vi "Create Mecanum Steering Frame.vi"(8 "error in (no error)":errorcluster, 9 "wheel separation length":dbl=1.5, 10 "wheel separation width":dbl=1.0, 11 "wheels":T1) -> (0 "error out":errorcluster, 3 "mecanum steering frame out":refnum<class "NI_Robotics_Mecanum Steering Frame.lvclass">)   [LabVIEW 2017, in "NI_Robotics_Mecanum Steering Frame.lvclass"]
doc: "Creates a steering frame of the type you specify. You must manually select the polymorphic instance to use."
uses:
  <vilib>/robotics/Steering/Mecanum Steering Frame/NI_Robotics_Mecanum Steering Frame.lvclass
  c:/Program Files (x86)/National Instruments/LabVIEW 2017/vi.lib/robotics/Steering/Steering Frame/NI_Robotics_Steering Frame.lvclass
  <vilib>/robotics/Steering/Mecanum Steering Frame/Mecanum Wheel Group.ctl
  <vilib>/robotics/Steering/Mecanum Wheel/NI_Robotics_Mecanum Wheel.lvclass
  c:/Program Files (x86)/National Instruments/LabVIEW 2017/vi.lib/robotics/Steering/Wheel/NI_Robotics_Wheel.lvclass
  <vilib>/robotics/Steering/Wheel/Rotation Direction.ctl
  <vilib>/robotics/Steering/Mecanum Wheel/Roller Orientation.ctl
  <vilib>/robotics/Steering/Mecanum Wheel/NI_Robotics_Mecanum Wheel.lvclass/NI_Robotics_Mecanum Wheel.ctl
  <vilib>/robotics/Steering/Wheel/NI_Robotics_Wheel.lvclass/NI_Robotics_Wheel.ctl
  <vilib>/robotics/Steering/Steering Frame/NI_Robotics_Steering Frame.lvclass/NI_Robotics_Steering Frame.ctl
  <vilib>/robotics/Steering/Mecanum Steering Frame/NI_Robotics_Mecanum Steering Frame.lvclass/NI_Robotics_Mecanum Steering Frame.ctl
  <vilib>/robotics/Steering/Wheel/Get Wheel Name.vi
  <vilib>/robotics/Steering/Wheel/Update Steering to Wheel Frame Transform.vi
  <vilib>/Analysis/coordinate.llb/Wrap Angle.vi
  <vilib>/Analysis/coordinate.llb/Wrap Angle (array).vi
  <vilib>/robotics/Steering/Wheel/NI_Robotics_Wheel.lvclass
  <vilib>/robotics/Steering/Steering Frame/NI_Robotics_Steering Frame.lvclass
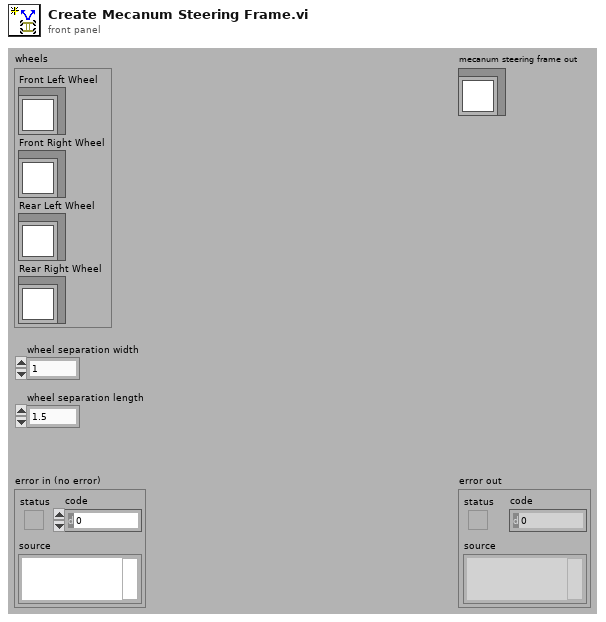
[diagram p1: front panel]
types:
  T1 = typedef "NI_Robotics_Mecanum Steering Frame.lvclass/Mecanum Wheel Group.ctl" = cluster{"Front Left Wheel":refnum<class "NI_Robotics_Mecanum Wheel.lvclass">, "Front Right Wheel":refnum<class "NI_Robotics_Mecanum Wheel.lvclass">, "Rear Left Wheel":refnum<class "NI_Robotics_Mecanum Wheel.lvclass">, "Rear Right Wheel":refnum<class "NI_Robotics_Mecanum Wheel.lvclass">}
  T2 = typedef "NI_Robotics_Mecanum Wheel.lvclass/Roller Orientation.ctl" = u16
  T3 = typedef "NI_Robotics_Wheel.lvclass/Rotation Direction.ctl" = u16
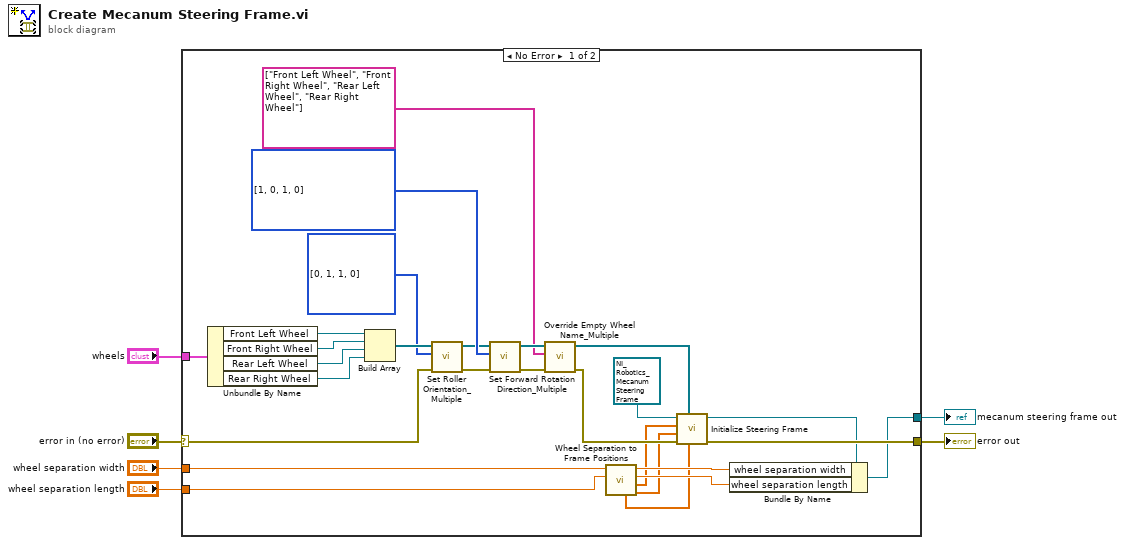
[diagram p0: block diagram]
diagram:
  n1 = case shown="No Error" "error in (no error)" {
    selector: "error in (no error)" -> [w18 w34]
    tunnel: [w32 w34] -> w5
    tunnel: [w14 _] -> w4
    tunnel: "wheel separation width" -> [w13 _]
    tunnel: "wheel separation length" -> [w12 _]
    tunnel: "wheels" -> [w31 _]
    frame No Error {
      w16 = T2[] [0, 1, 1, 0] items=["Left", "Right"] ("roller orientations")
      w26 = T3[] [1, 0, 1, 0] items=["Clockwise", "Counterclockwise"] ("Forward Rotation Directions")
      n2 = Unbundle By Name(w31) -> ("Front Left Wheel"=w30:refnum<class "NI_Robotics_Mecanum Wheel.lvclass">, "Front Right Wheel"=w29:refnum<class "NI_Robotics_Mecanum Wheel.lvclass">, "Rear Left Wheel"=w28:refnum<class "NI_Robotics_Mecanum Wheel.lvclass">, "Rear Right Wheel"=w27:refnum<class "NI_Robotics_Mecanum Wheel.lvclass">)
      n3 = Build Array(w30, w29, w28, w27) -> (w20:refnum<class "NI_Robotics_Mecanum Wheel.lvclass">[])
      n4 = call <vilib>:"Set Roller Orientation_Multiple.vi"("error in (no error)"=w18, "roller orientations"=w16, "mecanum wheels in"=w20) -> ("error out"=w17:errorcluster, "mecanum wheels out"=w19:refnum<class "NI_Robotics_Mecanum Wheel.lvclass">[])  [unwired: 7 in]
      n5 = call <vilib>:"Set Forward Rotation Direction_Multiple.vi"("error in (no error)"=w17, "forward rotation directions"=w26, "wheels in"=w19) -> ("error out"=w24:errorcluster, "wheels out"=w25:refnum<class "NI_Robotics_Wheel.lvclass">[])  [unwired: 7 in]
      n6 = call <vilib>:"Override Empty Wheel Name_Multiple.vi"("error in (no error)"=w24, "wheel names"=string[] ["Front Left Wheel", "Front Right Wheel", "Rear Left Wheel", "Rear Right Wheel"] ("Wheel IDs"), "wheels in"=w25) -> ("error out"=w23:errorcluster, "wheels out"=w21:refnum<class "NI_Robotics_Wheel.lvclass">[])  [unwired: 7 in]
      n7 = call <vilib>:"Wheel Separation to Frame Positions.vi"("wheel separation length"=w12, "wheel separation width"=w13) -> ("wheel y positions"=w8:dbl[], "wheel x positions"=w9:dbl[], "coerced wheel separation length"=w10:dbl, "coerced wheel separation width"=w11:dbl, "wheel frame angles (rad)"=w7:dbl[])  [unwired: 4 in, 1 out]
      n8 = call <vilib>:"Initialize Steering Frame.vi"("wheel frame angles (rad)"=w7, "wheels"=w21, "error in (no error)"=w23, "wheel y positions"=w8, "wheel x positions"=w9, "steering frame in"=refnum<class "NI_Robotics_Mecanum Steering Frame.lvclass"> refnum ("Mecanum Steering Frame in")) -> ("error out"=w32:errorcluster, "steering frame out"=w15:refnum<class "NI_Robotics_Mecanum Steering Frame.lvclass">)  [unwired: 4 in]
      n9 = Bundle By Name(cluster=w15, "wheel separation width"=w11, "wheel separation length"=w10) -> (w14:refnum<class "NI_Robotics_Mecanum Steering Frame.lvclass">)
    }
    frame Error {
    }
  }
  "error out" <- w5
  "mecanum steering frame out" <- w4
